vi "Get Kernel Time.vi"(8 "error in (no error) in":errorcluster, 11 "Action (Snap)":T1=enum."Snap") -> (0 "error out":errorcluster, 3 "Microseconds":u64)   [LabVIEW 2020]
uses:
  _Controls/Timer actions.ctl
  kernel32.dll
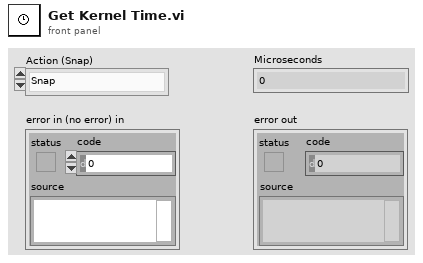
[diagram p1: front panel]
types:
  T1 = typedef "Timer actions.ctl" = enum16{"Reset", "Snap", "Total"}
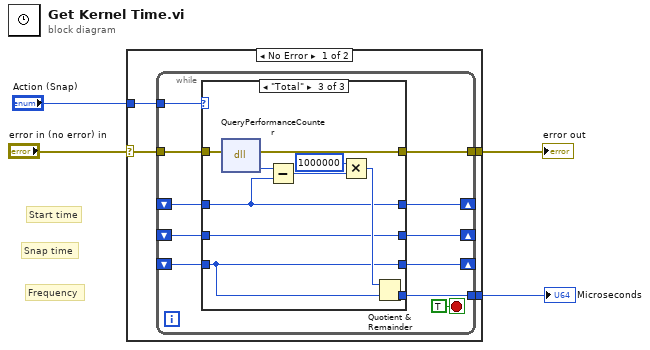
[diagram p0: block diagram]
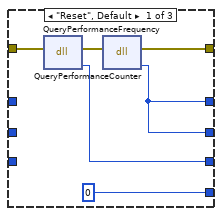
[diagram p2: hidden frame]
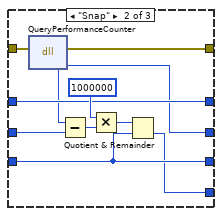
[diagram p3: hidden frame]
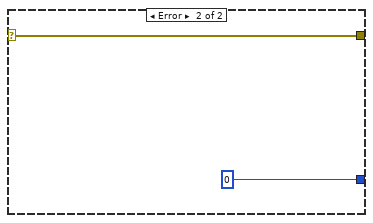
[diagram p4: hidden frame]
diagram:
  # "Snap time"
  # "Start time"
  # "Frequency"
  n1 = case shown="No Error" "error in (no error) in" {
    selector: "error in (no error) in" -> [w5 w47]
    tunnel: "Action (Snap)" -> [w8 _]
    tunnel: [w7 w47] -> w3
    tunnel: [w6 u64 0] -> w2
    frame No Error {
      n2 = while {
        tunnel: w8 -> [w19]
        shift-right: [w18] -> _
        shift-left: _ -> [w16]
        shift-right: [w15] -> _
        shift-left: _ -> [w14]
        tunnel: w5 -> [w13]
        tunnel: [w12] -> w7
        tunnel: [w11] -> w6
        shift-right: [w10] -> _
        shift-left: _ -> [w9]
        stop <- TRUE stop-if-true
        n3 = case shown="\"Total\"" w19 {
          tunnel: [w20 w27 w39] -> w18
          tunnel: w16 -> [_ w33 w39]
          tunnel: [w21 w29 w36] -> w15
          tunnel: w14 -> [_ w29 w36]
          tunnel: w13 -> [w25 w35 w42]
          tunnel: [w23 w34 w41] -> w12
          tunnel: [u64 0 w26 w38] -> w11
          tunnel: [w20 w28 w37] -> w10
          tunnel: w9 -> [_ w28 w37]
          frame "Reset", Default {
            n4 = dll-call lib="kernel32.dll" fn="QueryPerformanceFrequency"(error in=w25) -> (error out=w24:errorcluster, "lpFrequency"=w21:u64)  [unwired: 4 in, 1 out]
            n5 = dll-call lib="kernel32.dll" fn="QueryPerformanceCounter"(error in=w24) -> (error out=w23:errorcluster, "lpPerformanceCount"=w20:u64)  [unwired: 4 in, 1 out]
          }
          frame "Snap" {
            n6 = dll-call lib="kernel32.dll" fn="QueryPerformanceCounter"(error in=w35) -> (error out=w34:errorcluster, "lpPerformanceCount"=w27:u64)  [unwired: 4 in, 1 out]
            n7 = Subtract(x=w27, y=w33) -> (x-y=w32:u64)
            n8 = Multiply(x=u64 1000000, y=w32) -> (x*y=w30:u64)
            n9 = Quotient & Remainder(x=w30, y=w29) -> (floor(x/y)=w26:u64)  [unwired: 1 out]
          }
          frame "Total" {
            n10 = dll-call lib="kernel32.dll" fn="QueryPerformanceCounter"(error in=w42) -> (error out=w41:errorcluster, "lpPerformanceCount"=w40:u64)  [unwired: 4 in, 1 out]
            n11 = Subtract(x=w40, y=w37) -> (x-y=w45:u64)
            n12 = Multiply(x=u64 1000000, y=w45) -> (x*y=w43:u64)
            n13 = Quotient & Remainder(x=w43, y=w36) -> (floor(x/y)=w38:u64)  [unwired: 1 out]
          }
        }
      }
    }
    frame Error {
    }
  }
  "error out" <- w3
  "Microseconds" <- w2
